vi "Read To String Delimiter.vi"(8 "error in (no error)":errorcluster, 11 "Abs_Array in":refnum<class "Abs_Array.lvclass">) -> (0 "error out":errorcluster, 2 "To String Delimiter":string=",", 3 "Abs_Array out":refnum<class "Abs_Array.lvclass">)   [LabVIEW 2021, in "Abs_Array.lvclass"]
uses:
  Abs_Array.lvclass
  Abs_Array.lvclass/Abs_Array.ctl
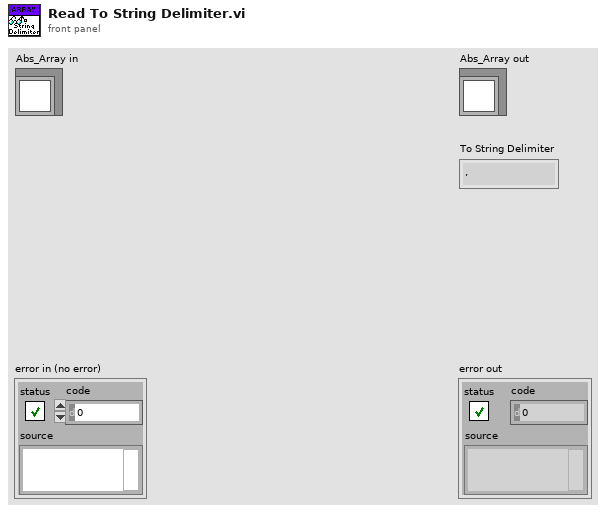
[diagram p1: front panel]
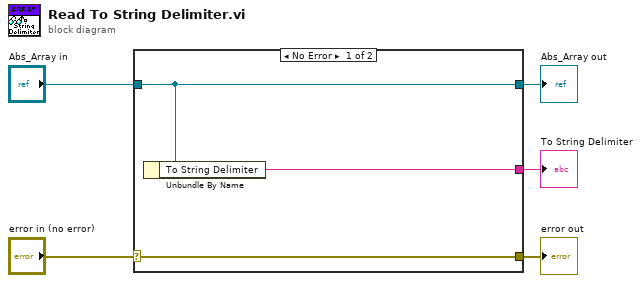
[diagram p0: block diagram]
diagram:
  n1 = case shown="No Error" "error in (no error)" {
    selector: "error in (no error)" -> [w8 w9]
    tunnel: [w8 w9] -> w4
    tunnel: [w7 w10] -> w2
    tunnel: "Abs_Array in" -> [w7 w10]
    tunnel: [w6 _] -> w1
    frame No Error {
      n2 = Unbundle By Name(w7) -> ("To String Delimiter"=w6:string)
    }
    frame Error {
    }
  }
  "error out" <- w4
  "Abs_Array out" <- w2
  "To String Delimiter" <- w1
